vi "16_11_dot_product.vi"(1 "B":fxp<+/-,16,11>[](array[numeric]), 2 "A":fxp<+/-,16,11>[](array[numeric])) -> (0 "c":fxp<+/-,16,11>)   [LabVIEW 2020]
panel:
  in  "accum":fxp<+/-,16,11> format="%#_32g"
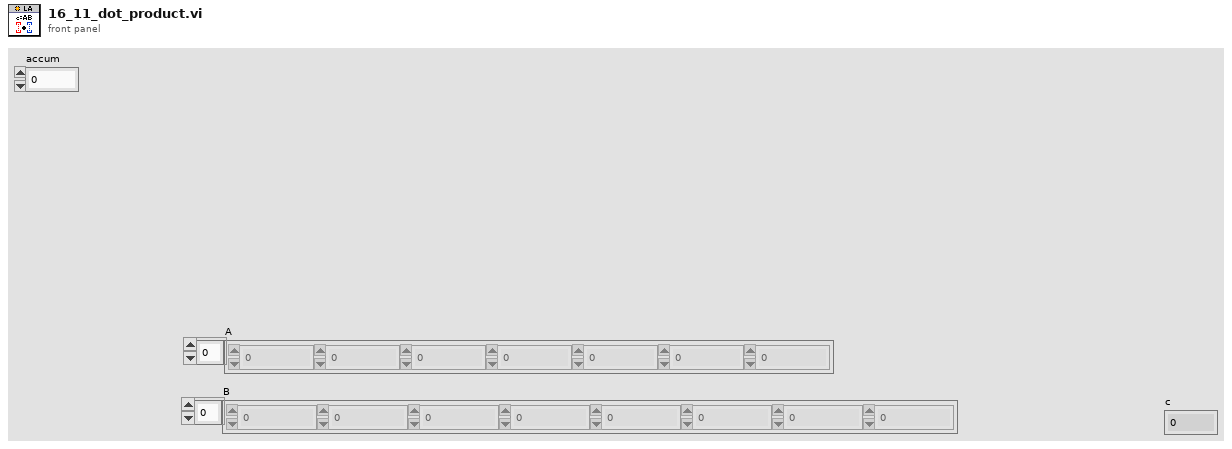
[diagram p1: front panel]
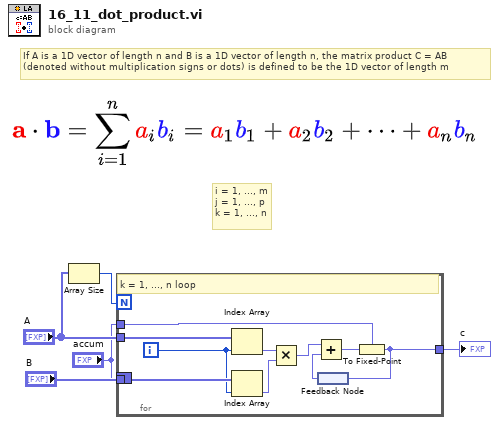
[diagram p0: block diagram]
diagram:
  # "If A is a 1D vector of length n and B is a 1D vector of length n, the matrix product C = AB \n(denoted without multiplication signs or dots) is defined to be the 1D vector of length m"
  # "i = 1, ..., m\nj = 1, ..., p\nk = 1, ..., n"
  n1 = Array Size(array="A") -> (size(s)=w2:i32)
  n2 = for {
    N: w2 -> [_]
    tunnel: "A" -> [w15]
    tunnel: "B" -> [w14]
    tunnel: [w6] -> w4
    border: "accum" -> [_]
    tunnel: "accum" -> [w7]
    i -> [w9]
    # "k = 1, ..., n loop"
    n3 = Index Array(array=w15, index=w9) -> (element=w13:fxp<+/-,16,11>)
    n4 = Index Array(array=w14, index=w9) -> (element=w12:fxp<+/-,16,11>)
    n5 = Multiply(x=w13, y=w12) -> (x*y=w11:fxp<+/-,32,22>)
    n6 = feedback #1() -> (w10:fxp<+/-,16,11>)
    n7 = Add(x=w11, y=w10) -> (x+y=w8:fxp<+/-,32,22>)
    n8 = To Fixed-Point(fixed-point type=w7, number=w8) -> (fixed-point=w6:fxp<+/-,16,11>)
    n9 = feedback-in #1(w6) -> ()
  }
  "c" <- w4
